vi "WPI_UltrasonicGetRange.vi"   [LabVIEW 2017]
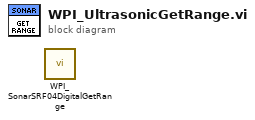
[diagram p0: block diagram]
diagram:
  n1 = call <vilib>:"WPI_SonarSRF04DigitalGetRange.vi"() -> ()  [unwired: 9 in, 3 out]
